vi "HTTP.vi"() -> ()   [LabVIEW 2017]
uses:
  <vilib>/daq.io/daq.io LabVIEW API/_typedefs/daqio-Credentials.ctl
  <vilib>/daq.io/daq.io LabVIEW API/_subs/daqio_Write_Single.vi
  <vilib>/daq.io/daq.io LabVIEW API/daqio minimal.lvlib
panel:
  in  "Stop Button":bool
  in  "登陸設定":T1
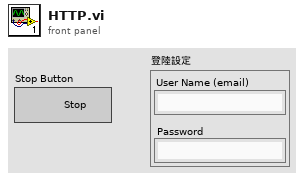
[diagram p1: front panel]
types:
  T1 = typedef "daqio minimal.lvlib/daqio-Credentials.ctl" = cluster{"User Name (email)":string, "Password":string}
  T2 = typedef "daqio minimal.lvlib/daqio-Type.ctl" = cluster{"daq.io ref":T3, "daq.io API Base":string, "Device Key":string, "Account ID":string, "online":bool, "SSL":bool, "buffer":bool}
  T3 = typedef "LabVIEWHTTPClient.lvlib/ClientHandle.ctl" = refnum<k1>
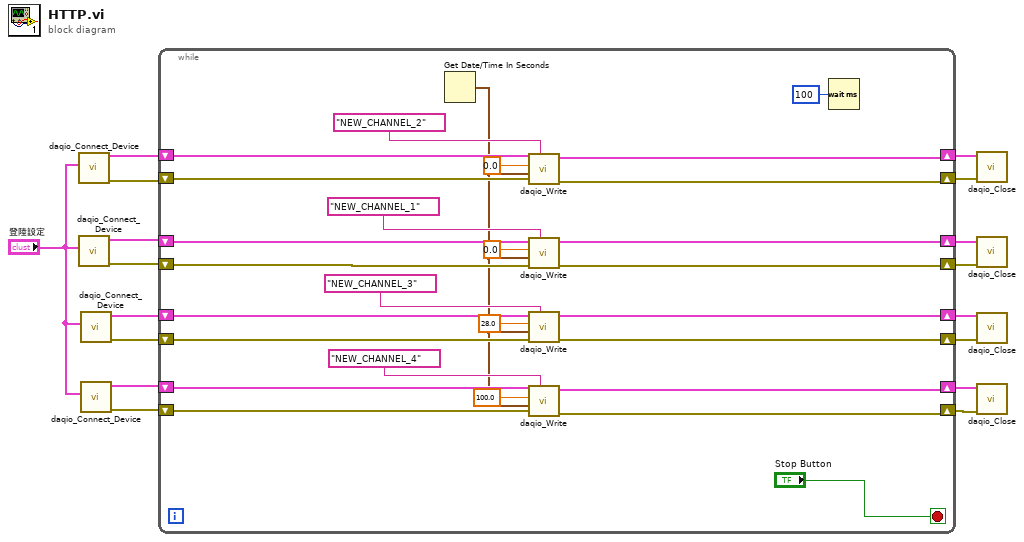
[diagram p0: block diagram]
diagram:
  n1 = call <vilib>:"daqio_Connect_Device.vi"("Credentials"="登陸設定") -> ("error out"=w15:errorcluster, "daq.io type out"=w16:T2)  [unwired: 8 in, 1 out]
  n2 = call <vilib>:"daqio_Connect_Device.vi"("Credentials"="登陸設定") -> ("error out"=w11:errorcluster, "daq.io type out"=w12:T2)  [unwired: 8 in, 1 out]
  n3 = call <vilib>:"daqio_Connect_Device.vi"("Credentials"="登陸設定") -> ("error out"=w13:errorcluster, "daq.io type out"=w14:T2)  [unwired: 8 in, 1 out]
  n4 = call <vilib>:"daqio_Connect_Device.vi"("Credentials"="登陸設定") -> ("error out"=w9:errorcluster, "daq.io type out"=w10:T2)  [unwired: 8 in, 1 out]
  n5 = while {
    shift-right: [w32] -> w8
    shift-left: w16 -> [w40]
    shift-right: [w31] -> w7
    shift-left: w15 -> [w39]
    shift-right: [w30] -> w6
    shift-left: w12 -> [w38]
    shift-right: [w29] -> w5
    shift-left: w11 -> [w37]
    shift-right: [w28] -> w4
    shift-left: w14 -> [w36]
    shift-right: [w27] -> w3
    shift-left: w13 -> [w35]
    shift-right: [w26] -> w2
    shift-left: w10 -> [w34]
    shift-right: [w25] -> w1
    shift-left: w9 -> [w33]
    stop <- "Stop Button" stop-if-true
    n6 = Get Date/Time In Seconds() -> (seconds since 1Jan1904=w23:timestamp)
    n7 = call-poly <vilib>:"daqio_Write.vi"("daq.io Device Channel Key"="NEW_CHANNEL_2", "error in (no error)"=w39, "timestamp"=w23, "value"=0.0, "daq.io type in"=w40) -> ("error out"=w31:errorcluster, "daq.io type out"=w32:T2)  [unwired: 5 in]
    n8 = call-poly <vilib>:"daqio_Write.vi"("daq.io Device Channel Key"="NEW_CHANNEL_1", "error in (no error)"=w37, "timestamp"=w23, "value"=0.0, "daq.io type in"=w38) -> ("error out"=w29:errorcluster, "daq.io type out"=w30:T2)  [unwired: 5 in]
    n9 = call-poly <vilib>:"daqio_Write.vi"("daq.io Device Channel Key"="NEW_CHANNEL_3", "error in (no error)"=w35, "timestamp"=w23, "value"=28.0, "daq.io type in"=w36) -> ("error out"=w27:errorcluster, "daq.io type out"=w28:T2)  [unwired: 5 in]
    n10 = call-poly <vilib>:"daqio_Write.vi"("daq.io Device Channel Key"="NEW_CHANNEL_4", "error in (no error)"=w33, "timestamp"=w23, "value"=100.0, "daq.io type in"=w34) -> ("error out"=w25:errorcluster, "daq.io type out"=w26:T2)  [unwired: 5 in]
    n11 = Wait (ms)(milliseconds to wait=u32 100) -> ()  [unwired: 1 out]
  }
  n12 = call <vilib>:"daqio_Close.vi"("error in (no error)"=w7, "daq.io type"=w8) -> ()  [unwired: 9 in, 1 out]
  n13 = call <vilib>:"daqio_Close.vi"("error in (no error)"=w5, "daq.io type"=w6) -> ()  [unwired: 9 in, 1 out]
  n14 = call <vilib>:"daqio_Close.vi"("error in (no error)"=w3, "daq.io type"=w4) -> ()  [unwired: 9 in, 1 out]
  n15 = call <vilib>:"daqio_Close.vi"("error in (no error)"=w1, "daq.io type"=w2) -> ()  [unwired: 9 in, 1 out]
